vi "DataLogger.vi"(0 "File Ref In":refnum<file>, 1 "Queue In":refnum<queue>, 2 "# Samples to Write":i32=50, 3 "Clear Error":bool=TRUE, 5 "Log State In":T1=enum."Rotate Log", 9 "String Path In":string, 11 "Error In":errorcluster, 12 "Channel Names In":string[](array[string]), 13 "File Path":string="C:\\work\\logs\\", 14 "File Name":string="FastData_") -> (4 "File Ref Out":refnum<file>, 6 "Log State Out":T1=enum."Rotate Log", 10 "String Path Out":string, 15 "Error Out":errorcluster)   [LabVIEW 2014]
uses:
  Controls/LogState.ctl
  <vilib>/Utility/file.llb/Write To Spreadsheet File (string).vi
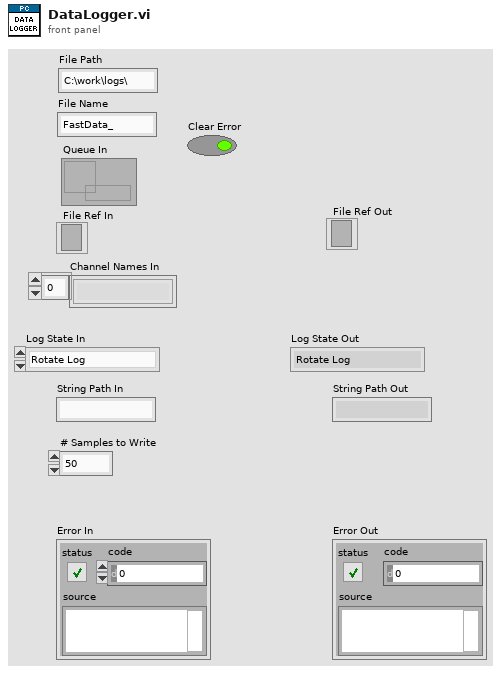
[diagram p1: front panel]
types:
  T1 = typedef "LogState.ctl" = enum16{"Remove Null Data", "Rotate Log", "Log Data", "Wait", "Close File", "Open File"}
  T2 = enum16{"open", "replace", "create", "open or create", "replace or create", "replace or create with confirmation"}
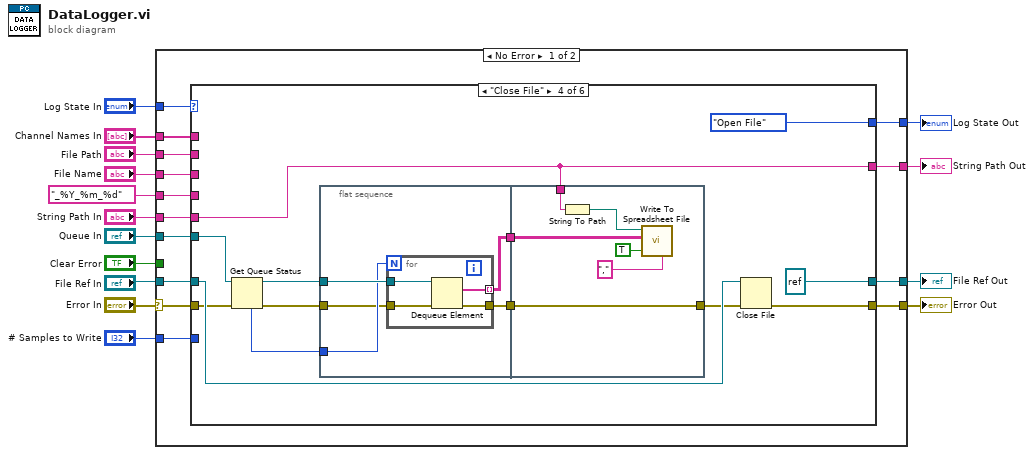
[diagram p0: block diagram]
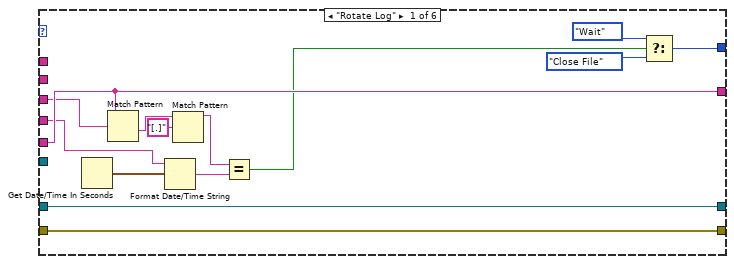
[diagram p2: hidden frame]
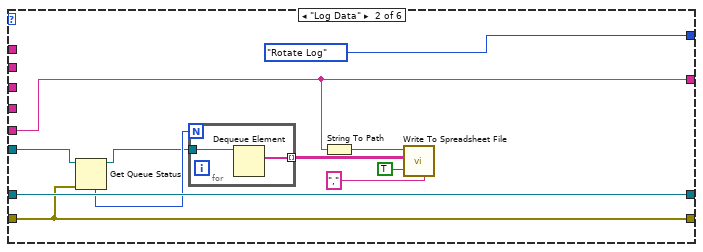
[diagram p3: hidden frame]
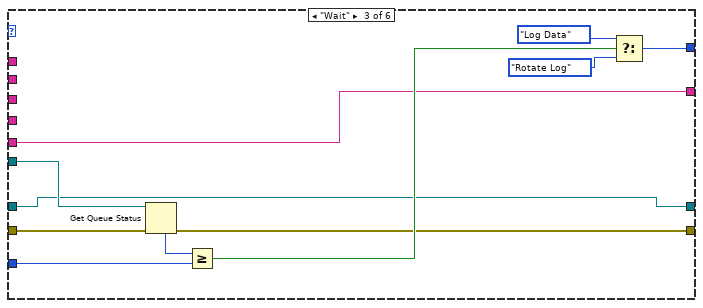
[diagram p4: hidden frame]
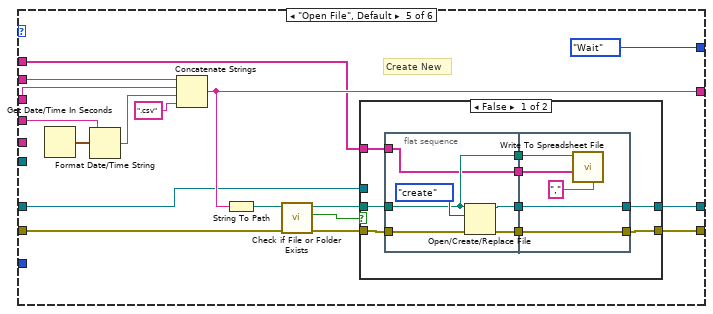
[diagram p5: hidden frame]
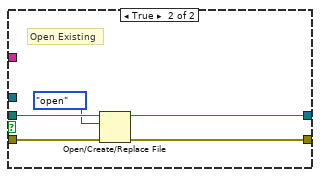
[diagram p6: hidden frame]
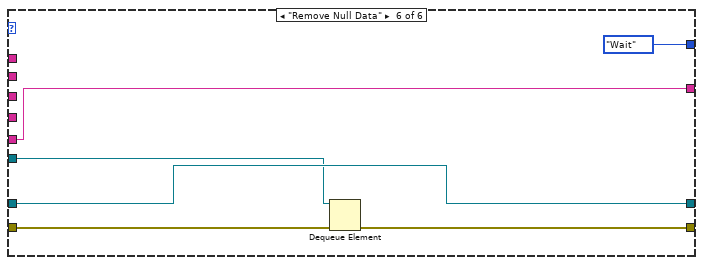
[diagram p7: hidden frame]
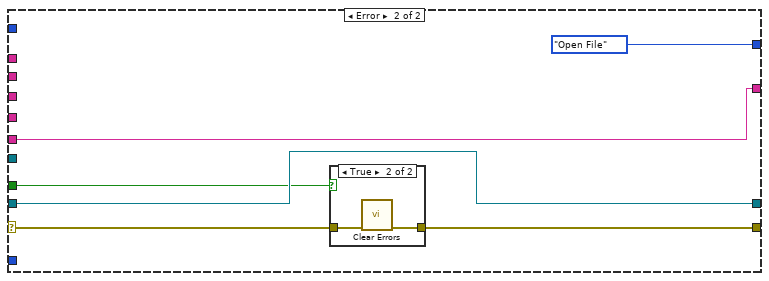
[diagram p8: hidden frame]
diagram:
  n1 = case shown="No Error" "Error In" {
    selector: "Error In" -> [w16 w148]
    tunnel: "String Path In" -> [w29 w146]
    tunnel: "Log State In" -> [w28 _]
    tunnel: [w27 w146] -> w13
    tunnel: [w26 w149] -> w12
    tunnel: [w25 LogState."Open File" ("Log State Out")] -> w11
    tunnel: "File Path" -> [w24 _]
    tunnel: "_%Y_%m_%d" ("time format string (%c)") -> [w23 _]
    tunnel: "File Name" -> [w22 _]
    tunnel: [w21 w145] -> w7
    tunnel: "File Ref In" -> [w20 w145]
    tunnel: "Queue In" -> [w19 _]
    tunnel: "# Samples to Write" -> [w18 _]
    tunnel: "Channel Names In" -> [w17 _]
    tunnel: "Clear Error" -> [_ w144]
    frame No Error {
      n2 = case shown="\"Close File\"" w28 {
        tunnel: w16 -> [w40 w47 w66 w76 w108 w140]
        tunnel: [w40 w47 w60 w79 w100 w139] -> w26
        tunnel: w19 -> [_ w45 w65 w69 _ w138]
        tunnel: [w43 LogState."Rotate Log" ("Log State") w64 LogState."Open File" ("Log State") LogState."Wait" ("Log State") LogState."Wait" ("Log State")] -> w25
        tunnel: [w39 w52 w59 w70 w107 w142] -> w27
        tunnel: w29 -> [w39 w52 w59 w70 _ w142]
        tunnel: w24 -> [_ _ _ _ w105 _]
        tunnel: w23 -> [w34 _ _ _ w106 _]
        tunnel: w22 -> [w31 _ _ _ w104 _]
        tunnel: [w30 w49 w58 refnum<file> refnum ("File Ref In") w97 w143] -> w21
        tunnel: w20 -> [w30 w49 w58 w77 w103 w143]
        tunnel: w17 -> [_ _ _ _ w98 _]
        tunnel: w18 -> [_ _ w57 _ _ _]
        frame "Rotate Log" {
          n3 = Get Date/Time In Seconds() -> (seconds since 1Jan1904=w36:timestamp)
          n4 = Match Pattern(string=w39, regular expression=w31) -> (after substring=w38:string)  [unwired: 1 in, 3 out]
          n5 = Format Date/Time String(time format string (%c)=w34, seconds (now)=w36) -> (date/time string=w33:string)  [unwired: 1 in]
          n6 = Match Pattern(string=w38, regular expression="[.]") -> (before substring=w32:string)  [unwired: 1 in, 3 out]
          n7 = Equal?(x=w32, y=w33) -> (x = y?=w35:bool)
          n8 = Select(t=LogState."Wait" ("Log State"), s=w35, f=LogState."Close File" ("Log State")) -> (s? t:f=w43:T1)
        }
        frame "Log Data" {
          n9 = Get Queue Status(queue=w45, error in (no error)=w47) -> (queue out=w44:refnum<queue>, # elements in queue=w46:i32)  [unwired: 1 in, 6 out]
          n10 = for {
            N: w46 -> [_]
            tunnel: w44 -> [w56]
            tunnel: [w55] -> w51 mode=indexing
            n11 = Dequeue Element(queue=w56) -> (element=w55:string[])  [unwired: 2 in, 3 out]
          }
          n12 = String To Path(string=w52) -> (path=w53:path)
          n13 = call-poly <vilib>:"Write To Spreadsheet File.vi"("delimiter (\\t)"="," ("delimiter (\\t)"), "append to file? (new file:F)"=TRUE, "2D data"=w51, "file path (dialog if empty)"=w53) -> ()  [unwired: 4 in, 1 out]
        }
        frame "Wait" {
          n14 = Get Queue Status(queue=w65, error in (no error)=w66) -> (error out=w60:errorcluster, # elements in queue=w67:i32)  [unwired: 1 in, 6 out]
          n15 = Greater Or Equal?(x=w67, y=w57) -> (x >= y?=w61:bool)
          n16 = Select(t=LogState."Log Data" ("Log State"), s=w61, f=LogState."Rotate Log" ("Log State")) -> (s? t:f=w64:T1)
        }
        frame "Close File" {
          n17 = Get Queue Status(queue=w69, error in (no error)=w76) -> (queue out=w68:refnum<queue>, error out=w74:errorcluster, # elements in queue=w75:i32)  [unwired: 1 in, 5 out]
          n18 = flat-sequence {
            tunnel: w68 -> [w84]
            tunnel: w75 -> [w83]
            tunnel: w74 -> [w82]
            tunnel: [w85] -> w72
            tunnel: [w81] -> w71
            tunnel: [w95] -> w73
            tunnel: w72 -> [w91]
            tunnel: w71 -> [w95]
            tunnel: w70 -> [w90]
            frame #0 {
              n19 = for {
                N: w83 -> [_]
                tunnel: w84 -> [w89]
                tunnel: [w88] -> w85 mode=indexing
                tunnel: [w87] -> w81
                tunnel: w82 -> [w86]
                n20 = Dequeue Element(queue=w89, error in (no error)=w86) -> (element=w88:string[], error out=w87:errorcluster)  [unwired: 1 in, 2 out]
              }
            }
            frame #1 {
              n21 = String To Path(string=w90) -> (path=w92:path)
              n22 = call-poly <vilib>:"Write To Spreadsheet File.vi"("delimiter (\\t)"="," ("delimiter (\\t)"), "append to file? (new file:F)"=TRUE, "2D data"=w91, "file path (dialog if empty)"=w92) -> ()  [unwired: 4 in, 1 out]
            }
          }
          n23 = Close File(refnum=w77, error in=w73) -> (error out=w79:errorcluster)  [unwired: 1 out]
        }
        frame "Open File", Default {
          # "Create New"
          n24 = Get Date/Time In Seconds() -> (seconds since 1Jan1904=w112:timestamp)
          n25 = Format Date/Time String(time format string (%c)=w106, seconds (now)=w112) -> (date/time string=w111:string)  [unwired: 1 in]
          n26 = Concatenate Strings(w105, w104, w111, ".csv" ("string")) -> (w107:string)
          n27 = String To Path(string=w107) -> (path=w110:path)
          n28 = call <vilib>:"Check if File or Folder Exists.vi"("error in (no error)"=w108, "path"=w110) -> ("error out"=w102:errorcluster, "file or folder exists?"=w101:bool, "dup path"=w99:path)  [unwired: 7 in]
          n29 = case shown="False" w101 {
            tunnel: w103 -> [_ _]
            tunnel: w102 -> [w121 w137]
            tunnel: [w119 w136] -> w100
            tunnel: w99 -> [w120 w135]
            tunnel: w98 -> [w115 _]
            tunnel: [w118 w133] -> w97
            frame False {
              n30 = flat-sequence {
                tunnel: w121 -> [w127]
                tunnel: w120 -> [w123]
                tunnel: [w125] -> w117
                tunnel: [w124] -> w116
                tunnel: w115 -> [w122]
                tunnel: [w123] -> w114
                tunnel: [w122] -> w113
                tunnel: [w131] -> w118
                tunnel: [w132] -> w119
                tunnel: w117 -> [w132]
                tunnel: w116 -> [w131]
                tunnel: w114 -> [w129]
                tunnel: w113 -> [w128]
                frame #0 {
                  n31 = Open/Create/Replace File(file path (use dialog)=w123, error in=w127, operation (0:open)=T2."create") -> (refnum out=w124:refnum<file>, error out=w125:errorcluster)  [unwired: 3 in, 1 out]
                }
                frame #1 {
                  n32 = call-poly <vilib>:"Write To Spreadsheet File.vi"("delimiter (\\t)"="," ("delimiter (\\t)"), "1D data"=w128, "file path (dialog if empty)"=w129) -> ()  [unwired: 5 in, 1 out]
                }
              }
            }
            frame True {
              # "Open Existing"
              n33 = Open/Create/Replace File(file path (use dialog)=w135, error in=w137, operation (0:open)=T2."open") -> (refnum out=w133:refnum<file>, error out=w136:errorcluster)  [unwired: 3 in, 1 out]
            }
          }
        }
        frame "Remove Null Data" {
          n34 = Dequeue Element(queue=w138, error in (no error)=w140) -> (error out=w139:errorcluster)  [unwired: 1 in, 3 out]
        }
      }
    }
    frame Error {
      n35 = case shown="True" w144 {
        tunnel: w148 -> [w150 w152]
        tunnel: [w150 w151] -> w149
        frame False {
        }
        frame True {
          n36 = call <vilib>:"Clear Errors.vi"("error in (no error)"=w152) -> ("error out"=w151:errorcluster)  [unwired: 5 in, 1 out]
        }
      }
    }
  }
  "String Path Out" <- w13
  "Error Out" <- w12
  "Log State Out" <- w11
  "File Ref Out" <- w7
